vi "Write Reg Patterns.vi"(10 "Reg Patterns":T1={"Write Reg Pattern"="C:\\Sandbox\\Supporting Materials\\Digital\\Compiled Patterns\\RFFE_RegWrite_Data.digipat", "Ext Write Reg Pattern"="C:\\Sandbox\\Supporting Materials\\Digital\\Compiled Patterns\\RFFE_RegWriteExt.digipat", "Cyc Ext Write Reg Pattern"="C:\\Sandbox\\Supporting Materials\\Digital\\Compiled Patterns\\RFFE_RegWriteExt_Cyc_Data.digipat", "Read Reg Pattern"="C:\\Sandbox\\Supporting Materials\\Digital\\Compiled Patterns\\RFFE_RegRead_Data.digipat"}, 11 "niDigital in":refnum<class "niDigital.lvclass">) -> (3 "niDigital out":refnum<class "niDigital.lvclass">)   [LabVIEW 2020, in "niDigital.lvclass"]
uses:
  niDigital.lvclass
  niDigital.lvclass/niDigital.ctl
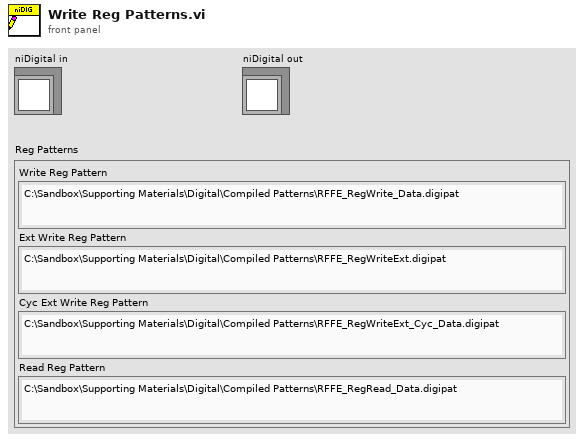
[diagram p1: front panel]
types:
  T1 = cluster{"Write Reg Pattern":string, "Ext Write Reg Pattern":string, "Cyc Ext Write Reg Pattern":string, "Read Reg Pattern":string}
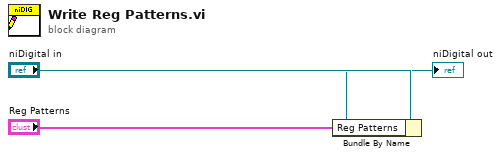
[diagram p0: block diagram]
diagram:
  n1 = Bundle By Name(cluster="niDigital in", "Reg Patterns"="Reg Patterns") -> (→"niDigital out":refnum<class "niDigital.lvclass">)
